vi "Calibration_concatenateMatrix.vi"(10 "Linear conversion Matrix2":dbl[][](array[numeric])=[[2.0, -2.0, 4.0], [2.0, 123.0, -4.1]], 11 "Linear conversion Matrix1":dbl[][](array[numeric])=[[1.0, 0.01, -1.0], [0.02123, 11.0, 0.1]]) -> (3 "concenated matrix":dbl[][](array[numeric])=[[1.95754, -21.98, 1.7999999999999998], [4.61129, 1353.02, 6.200000000000001]])   [LabVIEW 2011]
uses:
  <vilib>/Analysis/baseanly.llb/Real A x B.vi
  <vilib>/Analysis/NI_AALBase.lvlib
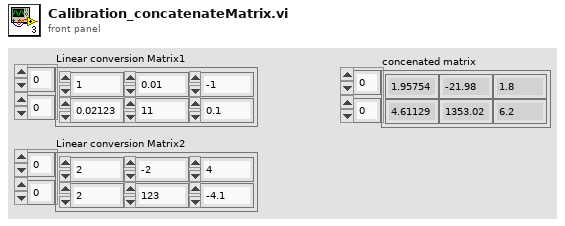
[diagram p1: front panel]
types:
  T1 = typedef "NI_Matrix.lvlib/RealMatrix.ctl" = dbl[][]
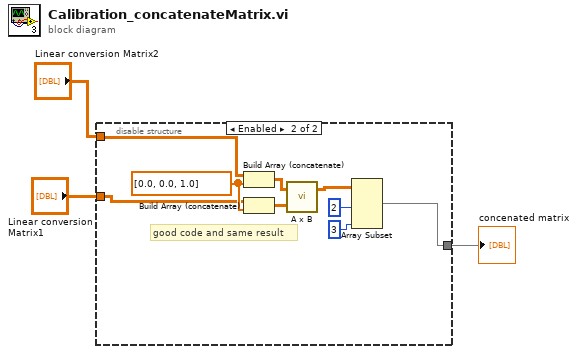
[diagram p0: block diagram]
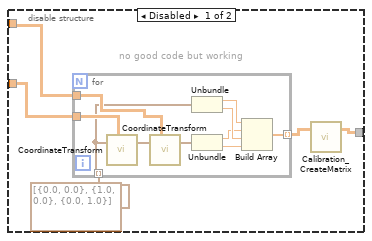
[diagram p2: hidden frame]
diagram:
  n1 = disable-structure shown="Enabled" {
    disable-tunnel: [w7 w19] -> w3
    disable-tunnel: "Linear conversion Matrix1" -> [w5 w21]
    disable-tunnel: "Linear conversion Matrix2" -> [w4 w20]
    frame Disabled {
      # "no good code but working"
      n2 = for {
        tunnel: cluster{dbl, dbl}[] [{0.0, 0.0}, {1.0, 0.0}, {0.0, 1.0}] ("sample points") -> [w11] mode=indexing
        tunnel: w5 -> [w18]
        tunnel: w4 -> [w16]
        tunnel: [w9] -> w6 mode=indexing
        n3 = call "CoordinateTransform.vi"("input coordiantes"=w11, "Conversion Matrix"=w18) -> ("output coordiantes"=w17:cluster{"x":dbl, "y":dbl})  [unwired: 2 in, 1 out]
        n4 = call "CoordinateTransform.vi"("input coordiantes"=w17, "Conversion Matrix"=w16) -> ("output coordiantes"=w10:cluster{"x":dbl, "y":dbl})  [unwired: 2 in, 1 out]
        n5 = Unbundle(w11) -> (w12:dbl, w14:dbl)
        n6 = Unbundle(w10) -> ("x"=w13:dbl, "y"=w15:dbl)
        n7 = Build Array(w12, w13, w14, w15) -> (w9:dbl[])
      }
      n8 = call "Calibration_CreateMatrix.vi"("CalibrationCoordinates: x,x',y,y'..."=w6) -> ("Linear conversion Matrix"=w7:dbl[][])  [unwired: 1 in, 1 out]
    }
    frame Enabled {
      w27 = dbl[] [0.0, 0.0, 1.0] ("appended v1")
      # "good code and same result"
      n9 = Build Array (concatenate)(w20, w27) -> (w23:dbl[][])
      n10 = Build Array (concatenate)(w21, w27) -> (w22:dbl[][])
      n11 = call-poly <vilib>:"A x B.vi"("B"=w22, "A"=w23) -> ("A x B"=w24:T1)  [unwired: 1 out]
      n12 = Array Subset(array=w24, length (row)=2 ("length"), length (col)=3 ("length")) -> (w19:T1)  [unwired: 2 in]
    }
  }
  "concenated matrix" <- w3
